vi "Check Item.vi"(6 "GObj Refnum":refnum<vi>, 8 "error in (no error)":errorcluster, 9 "VI Queue":refnum<queue>, 10 "New Result Event":refnum<user-event>, 11 "Search in":refnum<class "Search.lvclass">) -> (0 "error out":errorcluster, 3 "Search out":refnum<class "Search.lvclass">)   [LabVIEW 2020, in "Better Search.lvlib" / "Search.lvclass"]
uses:
  Search.lvclass
  BetterSearch/Search Result.ctl
  Search Result/Search Result.lvclass
  Better Search.lvlib
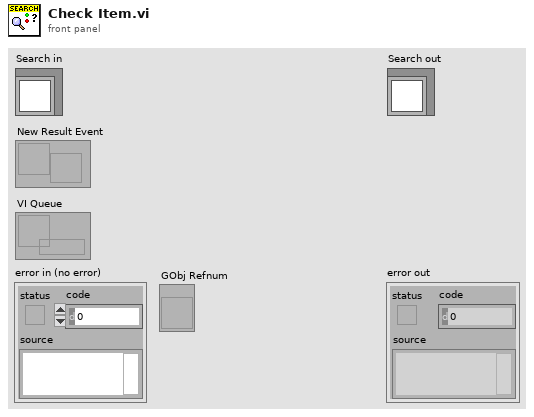
[diagram p1: front panel]
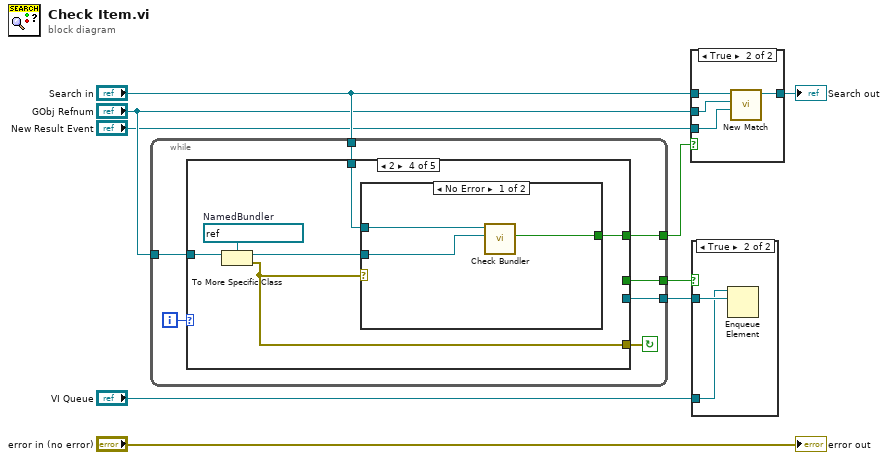
[diagram p0: block diagram]
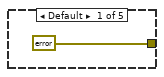
[diagram p4: hidden frame]
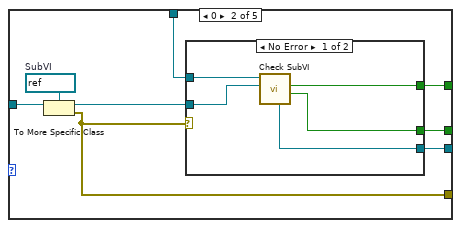
[diagram p5: hidden frame]
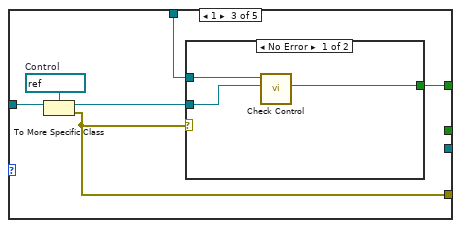
[diagram p7: hidden frame]
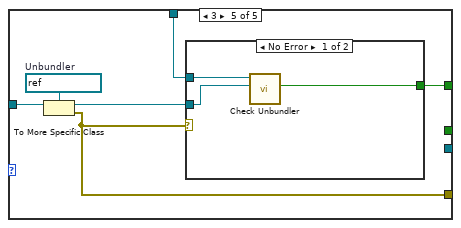
[diagram p10: hidden frame]
diagram:
  n1 = while {
    tunnel: "GObj Refnum" -> [w15]
    tunnel: [w14] -> w5
    tunnel: "Search in" -> [w13]
    tunnel: [w11] -> w3
    tunnel: [w10] -> w2
    i -> [w16]
    stop <- w12 continue-if-true
    n2 = case shown="2" w16 {
      tunnel: w15 -> [_ w25 w36 w45 w54]
      tunnel: [_ w20 w32 w41 w49] -> w14
      tunnel: w13 -> [_ w22 w33 w42 w51]
      tunnel: [errorcluster {"status"=FALSE, "code"=0, "source"=""} ("error out") w21 w31 w40 w50] -> w12
      tunnel: [_ w19 _ _ _] -> w11
      tunnel: [_ w18 _ _ _] -> w10
      frame Default {
      }
      frame 0 {
        w24 = refnum<vi> refnum  # SubVI
        n3 = To More Specific Class(target class=w24, reference=w25) -> (specific class reference=w23:refnum<vi>, error out=w21:errorcluster)  [unwired: 1 in]
        n4 = case shown="No Error" w21 {
          tunnel: w23 -> [w27 _]
          tunnel: w22 -> [w30 _]
          tunnel: [w29 _] -> w20
          tunnel: [w28 _] -> w19
          tunnel: [w26 _] -> w18
          frame No Error {
            n5 = call "Check SubVI.vi"("SubVI Refnum"=w27, "Search in"=w30) -> ("Add to Queue?"=w28:bool, "Match?"=w29:bool, "VI Refnum"=w26:refnum<vi>)  [unwired: 5 in, 2 out]
          }
          frame Error {
          }
        }
      }
      frame 1 {
        w35 = refnum<vi> refnum  # Control
        n6 = To More Specific Class(target class=w35, reference=w36) -> (specific class reference=w34:refnum<vi>, error out=w31:errorcluster)  [unwired: 1 in]
        n7 = case shown="No Error" w31 {
          tunnel: w34 -> [w38 _]
          tunnel: w33 -> [w39 _]
          tunnel: [w37 _] -> w32
          frame No Error {
            n8 = call "Check Control.vi"("Control"=w38, "Search in"=w39) -> ("Match?"=w37:bool)  [unwired: 7 in, 2 out]
          }
          frame Error {
          }
        }
      }
      frame 2 {
        w44 = refnum<vi> refnum  # NamedBundler
        n9 = To More Specific Class(target class=w44, reference=w45) -> (specific class reference=w43:refnum<vi>, error out=w40:errorcluster)  [unwired: 1 in]
        n10 = case shown="No Error" w40 {
          tunnel: w43 -> [w46 _]
          tunnel: w42 -> [w48 _]
          tunnel: [w47 _] -> w41
          frame No Error {
            n11 = call "Check Bundler.vi"("Bundler"=w46, "Search in"=w48) -> ("Match?"=w47:bool)  [unwired: 7 in, 2 out]
          }
          frame Error {
          }
        }
      }
      frame 3 {
        w53 = refnum<vi> refnum  # Unbundler
        n12 = To More Specific Class(target class=w53, reference=w54) -> (specific class reference=w52:refnum<vi>, error out=w50:errorcluster)  [unwired: 1 in]
        n13 = case shown="No Error" w50 {
          tunnel: w52 -> [w57 _]
          tunnel: w51 -> [w56 _]
          tunnel: [w55 _] -> w49
          frame No Error {
            n14 = call "Check Unbundler.vi"("Bundler"=w57, "Search in"=w56) -> ("Match?"=w55:bool)  [unwired: 7 in, 2 out]
          }
          frame Error {
          }
        }
      }
    }
  }
  n15 = case shown="True" w5 {
    tunnel: "Search in" -> [w58 w62]
    tunnel: "GObj Refnum" -> [_ w60]
    tunnel: "New Result Event" -> [_ w59]
    tunnel: [w58 w61] -> w4
    frame False {
    }
    frame True {
      n16 = call "New Match.vi"("New Result Event"=w59, "GObj Refnum"=w60, "Search in"=w62) -> ("Search out"=w61:refnum<class "Search.lvclass">)  [unwired: 7 in, 1 out]
    }
  }
  "Search out" <- w4
  n17 = case shown="True" w3 {
    tunnel: w2 -> [_ w64]
    tunnel: "VI Queue" -> [_ w63]
    frame False {
    }
    frame True {
      n18 = Enqueue Element(queue=w63, element=w64) -> ()  [unwired: 2 in, 3 out]
    }
  }
  "error out" <- "error in (no error)"
